vi "Test Load Virtual NEO480 cRIO XNET from EXCEL.vi"(11 "Test Case In":refnum<class "Test Instrument Manager.lvclass">) -> (0 "error out":errorcluster, 3 "Test Case Out":refnum<class "Test Instrument Manager.lvclass">)   [LabVIEW 2024, in "Test Instrument Manager.lvclass"]
uses:
  Test Instrument Manager.lvclass
  C:/Program Files/National Instruments/LabVIEW 2025/vi.lib/Astemes/LUnit/Test Case.lvclass
  Source/Interfaces/IRead Temperature/IRead Temperature.lvclass
  Source/Interfaces/IReadPressure/IRead Pressure.lvclass
  HAL/Source/Interfaces/IRead Dew Point/IRead Dew Point.lvclass
  Source/Interfaces/IVirtual Instrument/IVirtual Instrument.lvclass
  <vilib>/Astemes/LUnit/Test Case.lvclass/Test Case.ctl
  Test Instrument Manager.lvclass/Test Instrument Manager.ctl
  <vilib>/Astemes/LUnit/Test Case.lvclass
  Source/Instrument Manager/Instrument Manager.lvclass
panel:
  out "Dew Point":dbl
  out "Time Stamp d":timestamp format="%<%x %.3X>T"
  out "Time Stamp p":timestamp format="%<%x %.3X>T"
  out "Pressure":dbl
  out "iteration":bool
  out "Temperature":dbl format="%.2f °C"
  out "Time Stamp t":timestamp format="%<%x %.3X>T"
  in  "stop":bool
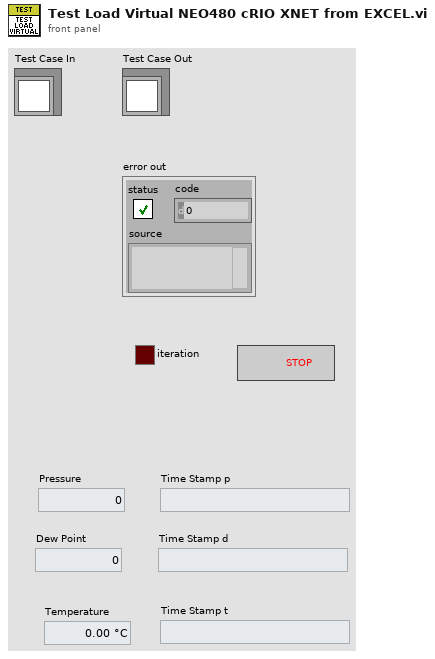
[diagram p1: front panel]
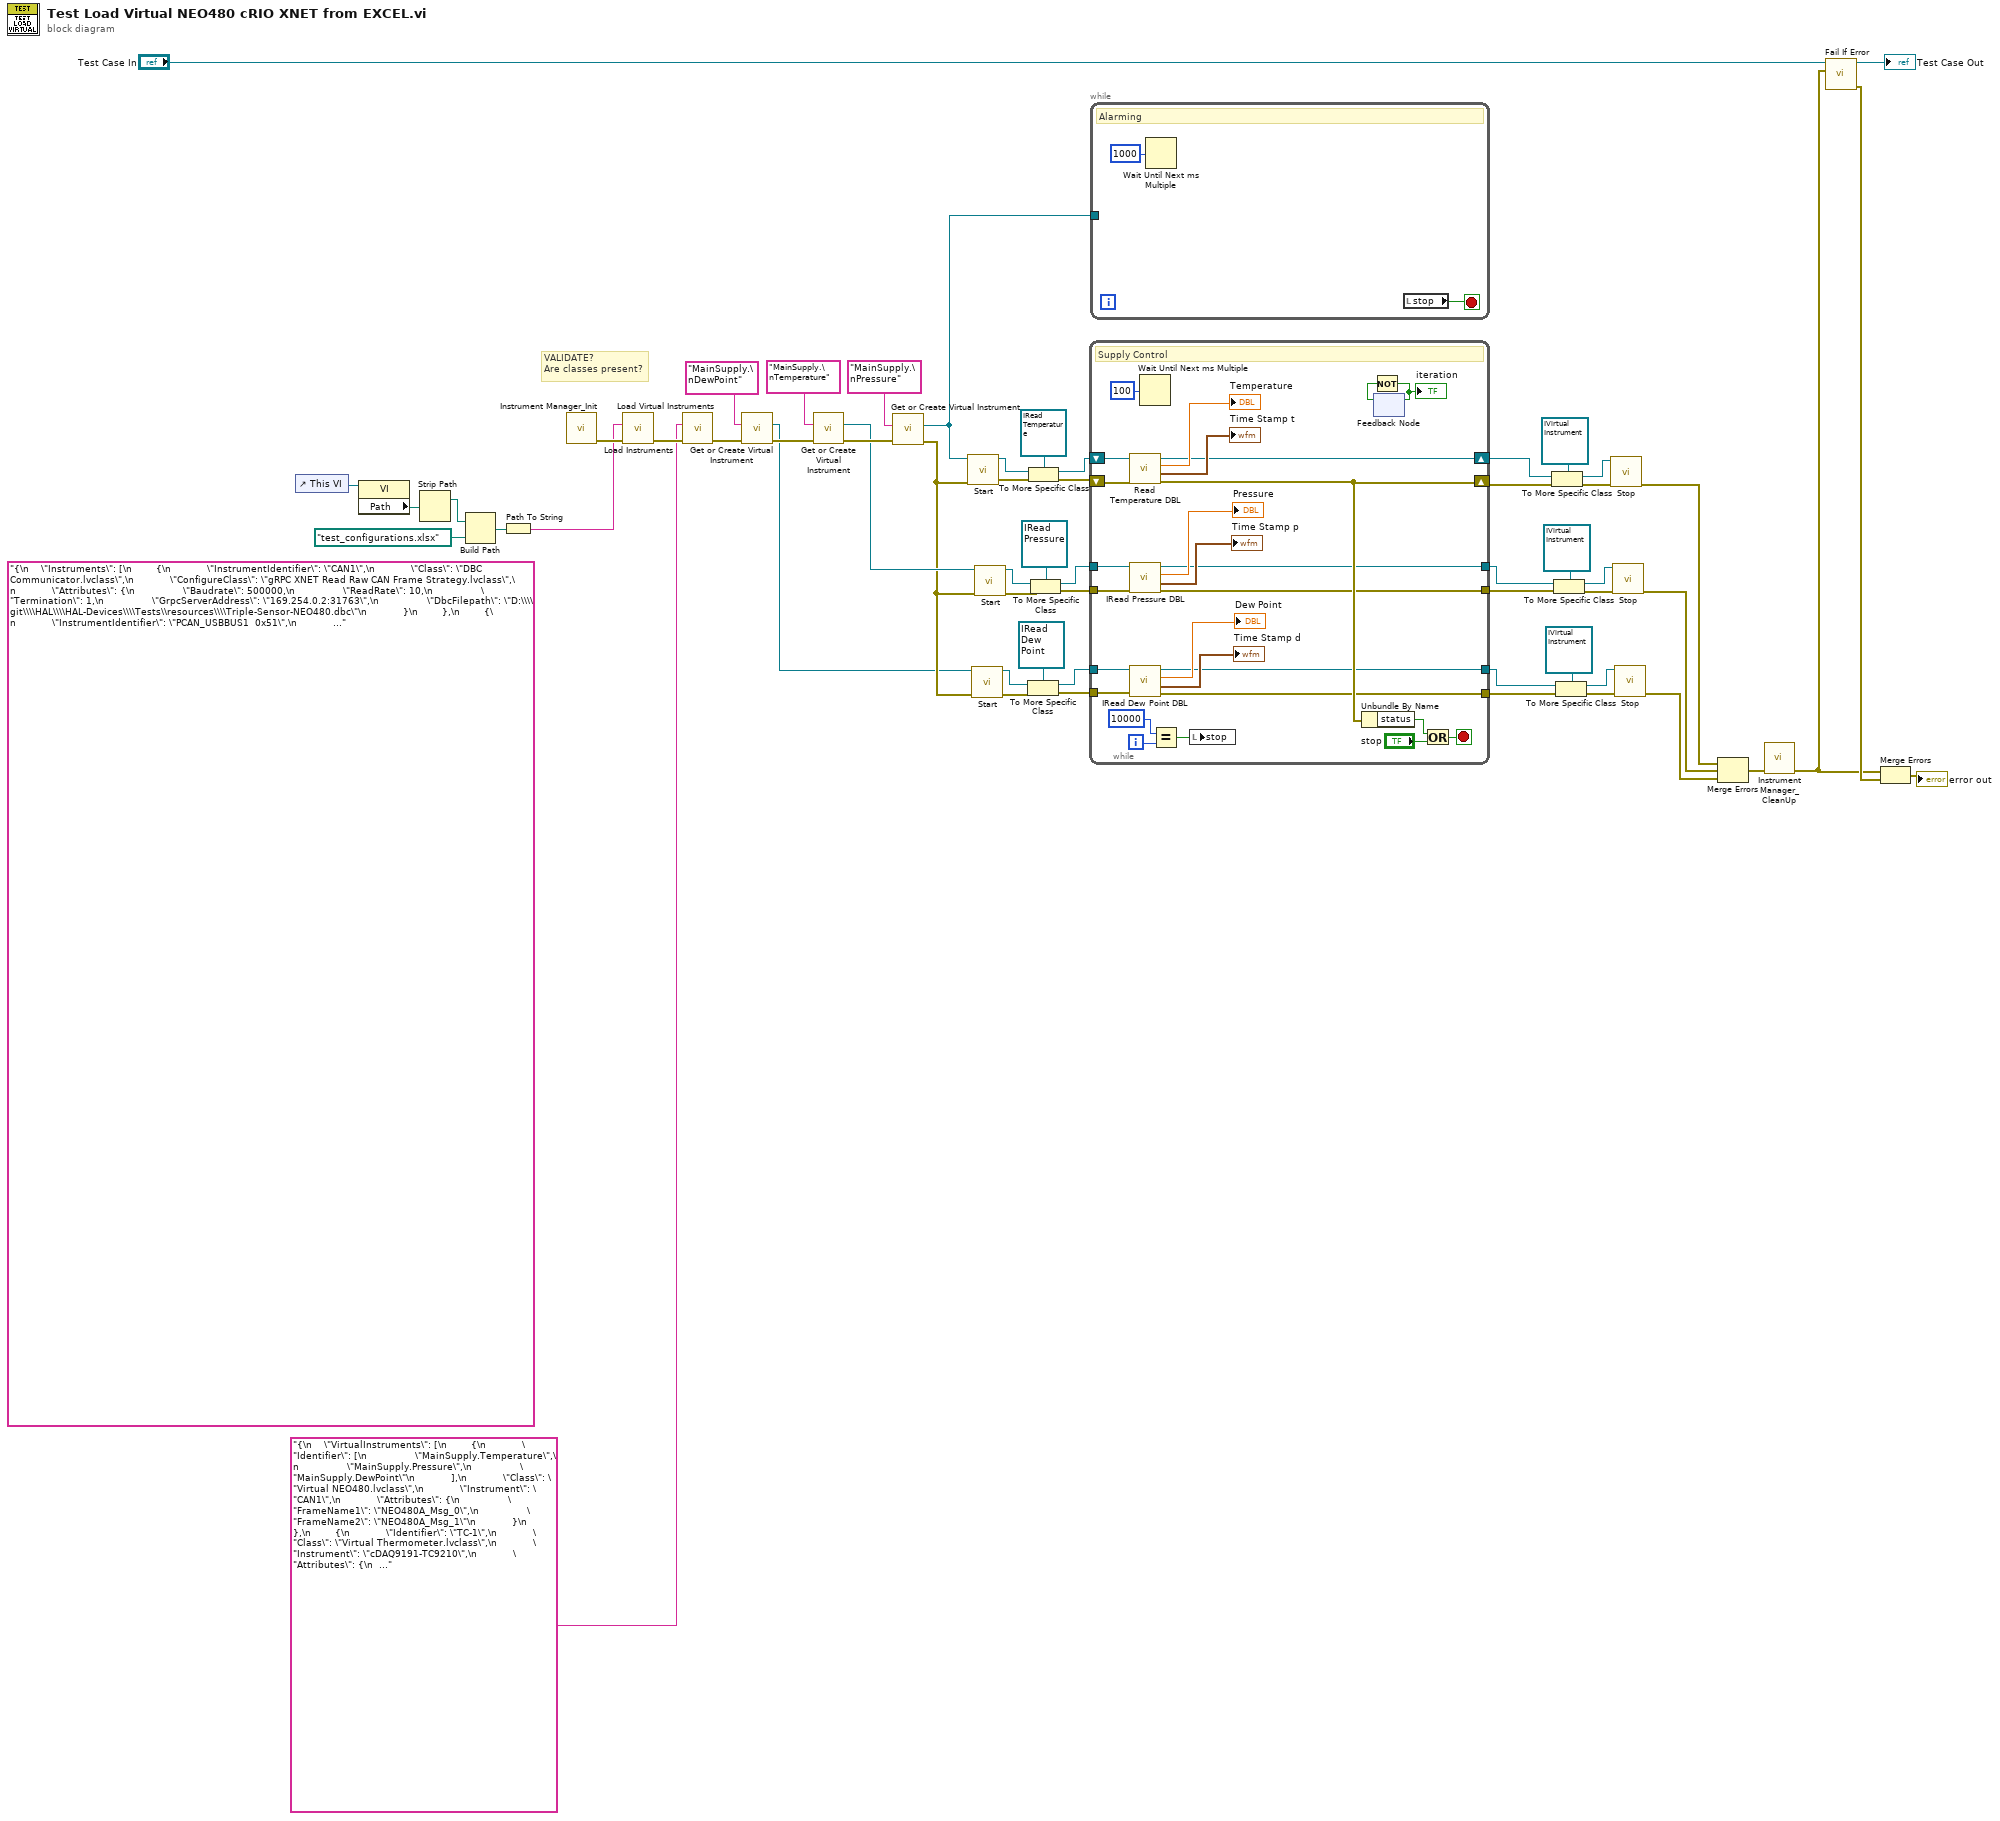
[diagram p0: block diagram]
diagram:
  (unwired) "{\n    \"Instruments\": [\n        {\n            \"InstrumentIdentifier\": \"CAN1\",\n            \"Class\": \"DBC Communicator.lvclass\",\n            \"ConfigureClass\": \"gRPC XNET Read Raw CAN Frame Strategy.lvclass\",\n            \"Attributes\": {\n                \"Baudrate\": 500000,\n                \"ReadRate\": 10,\n                \"Termination\": 1,\n                \"GrpcServerAddress\": \"169.254.0.2:31763\",\n                \"DbcFilepath\": \"D:\\\\git\\\\HAL\\\\HAL-Devices\\\\Tests\\resources\\\\Triple-Sensor-NEO480.dbc\"\n            }\n        },\n        {\n            \"InstrumentIdentifier\": \"PCAN_USBBUS1  0x51\",\n            \"Class\": \"DBC Communicator.lvclass\",\n            \"ConfigureClass\": \"PCAN Read Raw CAN Frame Strategy.lvclass\",\n            \"Attributes\": {\n                \"Baudrate\": 500000,\n                \"ReadRate\": 10,\n                \"DbcFilepath\": \"D:\\\\git\\\\HAL\\\\HAL-Devices\\\\Tests\\resources\\\\Triple-Sensor-NEO480.dbc\"\n            }\n        },\n        {\n            \"InstrumentIdentifier\": \"cDAQ9191-TC9210\",\n            \"Class\": \"Thermometer Multichannel.lvclass\",\n            \"ConfigureClass\": \"DAQmx Thermocouple Continuous Read Strategy.lvclass\",\n            \"Attributes\": {\n                \"ReadRate\": 10,\n                \"Channels\": [\n                    {\n                        \"Name\": \"ai0\",\n                        \"Enabled\": true,\n                        \"MinimumValue\": 0,\n                        \"MaximumValue\": 100,\n                        \"ThermocoupleType\": \"J\",\n                        \"Units\": \"Deg C\",\n                        \"CjcChannel\": \"\",\n                        \"CjcSource\": \"Constant Value\",\n                        \"CjcValue\": 25\n                    }\n                ],\n                \"Timing\": {\n                    \"Type\": \"Sample Clock\",\n                    \"SamplesPerChannel\": 1000,\n                    \"SampleMode\": \"Continuous Samples\",\n                    \"SampleRate\": 10,\n                    \"SampleClockSource\": \"OnboardClock\",\n                    \"ActiveEdge\": \"Rising\"\n                },\n                \"Trigger\": {\n                    \"TriggerType\": \"No Trigger\"\n                }\n            }\n        }\n    ]\n}" ("Source")
  # "VALIDATE?\nAre classes present?"
  n1 = control-ref of="This VI"() -> (w6:refnum<vi>)
  n2 = property class="VI"(reference=w6) -> ("Path"=w5:path)  [unwired: 1 in, 2 out]
  n3 = Strip Path(path=w5) -> (stripped path=w4:path)  [unwired: 1 out]
  n4 = Build Path(base path=w4, name or relative path=path "test_configurations.xlsx") -> (appended path=w2:path)
  n5 = Path To String(path=w2) -> (string=w1:string)
  n6 = call "Instrument Manager_Init.vi"() -> ("Error Out"=w53:errorcluster)  [unwired: 10 in, 1 out]
  n7 = call "Load Instruments.vi"("Error In"=w53, "Source"=w1) -> ("Error Out"=w50:errorcluster)  [unwired: 9 in]
  n8 = call "Load Virtual Instruments.vi"("Error In"=w50, "Source"="{\n    \"VirtualInstruments\": [\n        {\n            \"Identifier\": [\n                \"MainSupply.Temperature\",\n                \"MainSupply.Pressure\",\n                \"MainSupply.DewPoint\"\n            ],\n            \"Class\": \"Virtual NEO480.lvclass\",\n            \"Instrument\": \"CAN1\",\n            \"Attributes\": {\n                \"FrameName1\": \"NEO480A_Msg_0\",\n                \"FrameName2\": \"NEO480A_Msg_1\"\n            }\n        },\n        {\n            \"Identifier\": \"TC-1\",\n            \"Class\": \"Virtual Thermometer.lvclass\",\n            \"Instrument\": \"cDAQ9191-TC9210\",\n            \"Attributes\": {\n                \"Channel\": \"ai0\"\n            }\n        }\n    ]\n}") -> ("Error Out"=w21:errorcluster)  [unwired: 9 in]
  n9 = call "Get or Create Virtual Instrument.vi"("Error In"=w21, "Virtual Instrument Identifier"="MainSupply.\nDewPoint" ("Instrument Identifier")) -> ("Error Out"=w20:errorcluster, "IVritual Instrument"=w16:refnum<class "IVirtual Instrument.lvclass">)  [unwired: 8 in]
  n10 = call "Get or Create Virtual Instrument.vi"("Error In"=w20, "Virtual Instrument Identifier"="MainSupply.\nTemperature") -> ("Error Out"=w48:errorcluster, "IVritual Instrument"=w23:refnum<class "IVirtual Instrument.lvclass">)  [unwired: 8 in]
  n11 = call "Get or Create Virtual Instrument.vi"("Error In"=w48, "Virtual Instrument Identifier"="MainSupply.\nPressure" ("Instrument Identifier")) -> ("Error Out"=w22:errorcluster, "IVritual Instrument"=w7:refnum<class "IVirtual Instrument.lvclass">)  [unwired: 8 in]
  n12 = call-dynamic "Start.vi"("error in"=w22, "IRunnable in"=w7) -> ("error out"=w41:errorcluster, "IRunnable out"=w42:refnum<class "IVirtual Instrument.lvclass">)  [unwired: 8 in]
  n13 = call-dynamic "Start.vi"("error in"=w22, "IRunnable in"=w16) -> ("error out"=w28:errorcluster, "IRunnable out"=w29:refnum<class "IVirtual Instrument.lvclass">)  [unwired: 8 in]
  n14 = call-dynamic "Start.vi"("error in"=w22, "IRunnable in"=w23) -> ("error out"=w38:errorcluster, "IRunnable out"=w37:refnum<class "IVirtual Instrument.lvclass">)  [unwired: 8 in]
  n15 = To More Specific Class(target class=refnum<class "IRead Dew Point.lvclass"> refnum ("IRead Dew Point.lvclass"), reference=w29, error in=w28) -> (specific class reference=w26:refnum<class "IRead Dew Point.lvclass">, error out=w27:errorcluster)
  n16 = To More Specific Class(target class=refnum<class "IRead Temperature.lvclass"> refnum ("IRead Temperature.lvclass"), reference=w42, error in=w41) -> (specific class reference=w39:refnum<class "IRead Temperature.lvclass">, error out=w40:errorcluster)
  n17 = To More Specific Class(target class=refnum<class "IRead Pressure.lvclass"> refnum ("IRead Pressure.lvclass"), reference=w37, error in=w38) -> (specific class reference=w25:refnum<class "IRead Pressure.lvclass">, error out=w24:errorcluster)
  n18 = while {
    shift-right: [w76] -> w46
    shift-left: w39 -> [w72]
    shift-right: [w77] -> w55
    shift-left: w40 -> [w73]
    tunnel: w27 -> [w66]
    tunnel: w26 -> [w65]
    tunnel: w25 -> [w64]
    tunnel: w24 -> [w63]
    tunnel: [w62] -> w9
    tunnel: [w61] -> w10
    tunnel: [w60] -> w11
    tunnel: [w59] -> w12
    i -> [w81]
    stop <- w82 stop-if-true
    # "Supply Control"
    n19 = call-dynamic "Read Temperature DBL.vi"("error in"=w73, "IRead Temperature in"=w72) -> ("error out"=w77:errorcluster, "Time Stamp"=→"Time Stamp t":timestamp, "Temperature"=→"Temperature":dbl, "IRead Temperature out"=w76:refnum<class "IRead Temperature.lvclass">)  [unwired: 6 in]
    n20 = call-dynamic "IRead Pressure DBL.vi"("error in"=w63, "IRead Pressure in"=w64) -> ("error out"=w62:errorcluster, "Time Stamp"=→"Time Stamp p":timestamp, "Pressure"=→"Pressure":dbl, "IRead Pressure out"=w61:refnum<class "IRead Pressure.lvclass">)  [unwired: 6 in]
    n21 = call-dynamic "IRead Dew Point DBL.vi"("error in"=w66, "IRead Dew Point in"=w65) -> ("error out"=w59:errorcluster, "Time Stamp"=→"Time Stamp d":timestamp, "Dew Point"=→"Dew Point":dbl, "IRead Dew Point out"=w60:refnum<class "IRead Dew Point.lvclass">)  [unwired: 6 in]
    n22 = Wait Until Next ms Multiple(millisecond multiple=u32 100) -> ()  [unwired: 1 out]
    n23 = Equal?(x=10000, y=w81) -> (x = y?=w71:bool)
    n24 = local write "stop"(w71) -> ()
    n25 = Unbundle By Name(w77) -> ("status"=w78:bool)
    n26 = feedback #1() -> (w75:bool)  [unwired: 1 in]
    n27 = Not(x=w75) -> (.not. x?=w74:bool)
    "iteration" <- w74
    n28 = feedback-in #1(w74) -> ()
    n29 = Or(x=w78, y="stop") -> (x .or. y?=w82:bool)
  }
  n30 = while {
    tunnel: w7 -> [_]
    stop <- w86 stop-if-true
    # "Alarming"
    n31 = Wait Until Next ms Multiple(millisecond multiple=u32 1000) -> ()  [unwired: 1 out]
    n32 = local read "stop"() -> (w86:bool)
  }
  n33 = To More Specific Class(target class=refnum<class "IVirtual Instrument.lvclass"> refnum ("IVirtual Instrument.lvclass"), reference=w46, error in=w55) -> (specific class reference=w44:refnum<class "IVirtual Instrument.lvclass">, error out=w47:errorcluster)
  n34 = To More Specific Class(target class=refnum<class "IVirtual Instrument.lvclass"> refnum ("IVirtual Instrument.lvclass"), reference=w10, error in=w9) -> (specific class reference=w35:refnum<class "IVirtual Instrument.lvclass">, error out=w33:errorcluster)
  n35 = To More Specific Class(target class=refnum<class "IVirtual Instrument.lvclass"> refnum ("IVirtual Instrument.lvclass"), reference=w11, error in=w12) -> (specific class reference=w13:refnum<class "IVirtual Instrument.lvclass">, error out=w15:errorcluster)
  n36 = call-dynamic "Stop.vi"("error in"=w47, "IRunnable in"=w44) -> ("error out"=w52:errorcluster)  [unwired: 8 in, 1 out]
  n37 = call-dynamic "Stop.vi"("error in"=w33, "IRunnable in"=w35) -> ("error out"=w31:errorcluster)  [unwired: 8 in, 1 out]
  n38 = call-dynamic "Stop.vi"("error in"=w15, "IRunnable in"=w13) -> ("error out"=w8:errorcluster)  [unwired: 8 in, 1 out]
  n39 = Merge Errors(w52, w31, w8) -> (w32:errorcluster)
  n40 = call "Instrument Manager_CleanUp.vi"("Error In"=w32) -> ("Error Out"=w51:errorcluster)  [unwired: 10 in]
  n41 = call <vilib>:"Fail If Error.vi"("Assert error"=w51, "LUnit Test Case In"="Test Case In") -> ("error out"=w56:errorcluster, "LUnit Test Case Out"=→"Test Case Out":refnum<class "Test Instrument Manager.lvclass">)  [unwired: 8 in]
  n42 = Merge Errors(w51, w56) -> (→"error out":errorcluster)
